vi "FLEnergySet.vi"(8 "Error In":errorcluster, 9 "Energy (J)":dbl=2.34 min=2.34 max=4.7 step=0.01 format="%_3g", 10 "delay before read (ms)":u32=500, 11 "VISA resource name":refnum<visa-resource-name>) -> (0 "Error Out":errorcluster, 1 "Write byte count":u32, 2 "Read byte count":u32, 3 "read buffer":string)   [LabVIEW 2016]
uses:
  <vilib>/Instr/_visa.llb/VISA Configure Serial Port (Instr).vi
panel:
  out "Bytes read":u32
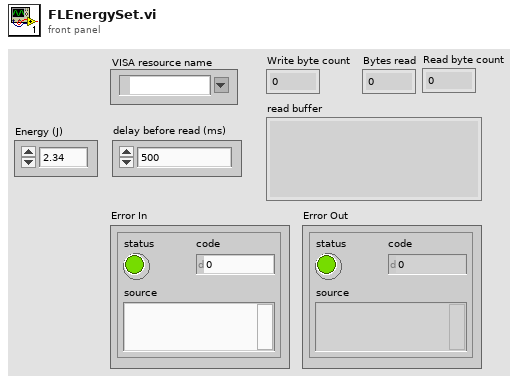
[diagram p1: front panel]
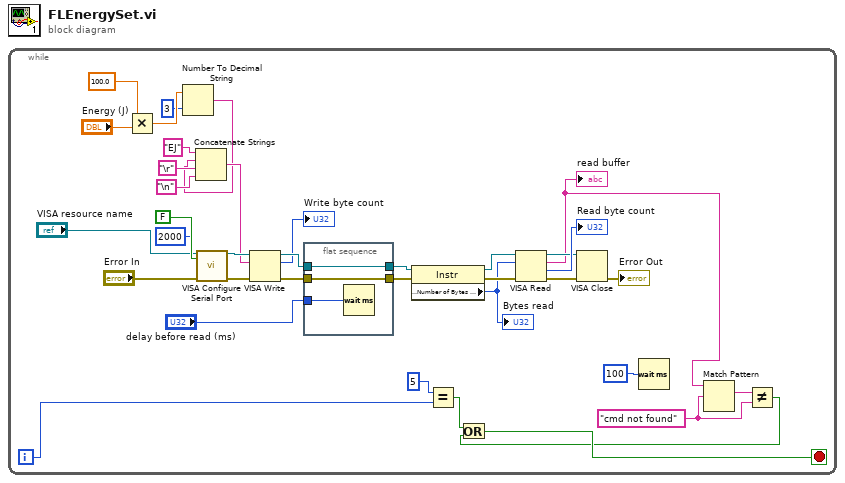
[diagram p0: block diagram]
diagram:
  n1 = while {
    i -> [w1]
    stop <- w3 stop-if-true
    w7 = "cmd not found" ("regular expression")
    n2 = Multiply(x=100.0, y="Energy (J)") -> (x*y=w13:dbl)
    n3 = Number To Decimal String(number=w13, width (-)=i16 3) -> (decimal integer string=w10:string)
    n4 = Concatenate Strings("EJ" ("Command"), w10, "\r", "\n") -> (w30:string)
    n5 = call-poly "VISA Configure Serial Port"("VISA resource name"="VISA resource name", "timeout (10sec)"=u32 2000, "Enable Termination\nChar (T)"=FALSE ("Enable Termination\nChar (T)"), "error in (no error)"="Error In") -> ("VISA resource name out"=w31:refnum<visa-resource-name>, "error out"=w29:errorcluster)  [unwired: 5 in, 5 out]
    n6 = VISA Write(VISA resource name=w31, write buffer=w30, error in (no error)=w29) -> (VISA resource name out=w27:refnum<visa-resource-name>, return count=→"Write byte count":u32, error out=w26:errorcluster)
    n7 = flat-sequence {
      tunnel: w26 -> [w39]
      tunnel: [w39] -> w24
      tunnel: w27 -> [w38]
      tunnel: [w38] -> w23
      tunnel: "delay before read (ms)" -> [w40]
      frame #0 {
        n8 = Wait (ms)(milliseconds to wait=w40) -> ()  [unwired: 1 out]
      }
    }
    n9 = property class="Instr"(reference=w23, error in=w24) -> (reference out=w19:refnum<visa-resource-name>, error out=w18:errorcluster, "Serial Settings:Number of Bytes at Serial Port"=w17:u32)
    "Bytes read" <- w17
    n10 = Equal?(x=5, y=w1) -> (x = y?=w4:bool)
    n11 = VISA Read(VISA resource name=w19, byte count=w17, error in (no error)=w18) -> (VISA resource name out=w21:refnum<visa-resource-name>, read buffer=w6:string, return count=→"Read byte count":u32, error out=w20:errorcluster)
    "read buffer" <- w6
    n12 = VISA Close(VISA resource name=w21, error in (no error)=w20) -> (error out=→"Error Out":errorcluster)
    n13 = Wait (ms)(milliseconds to wait=u32 100) -> ()  [unwired: 1 out]
    n14 = Match Pattern(string=w6, regular expression=w7) -> (match substring=w8:string)  [unwired: 1 in, 3 out]
    n15 = Not Equal?(x=w8, y=w7) -> (x != y?=w2:bool)
    n16 = Or(x=w4, y=w2) -> (x .or. y?=w3:bool)
  }
